vi "Dijkstra.vi"(2 "error in (no error)":errorcluster, 4 "Edges":T1(array[cluster]), 5 "Number of Nodes":i32) -> (0 "error out":errorcluster, 1 "Path":i32[](array[numeric]))   [LabVIEW 2009]
panel:
  out "appended array":dbl[](array[numeric])
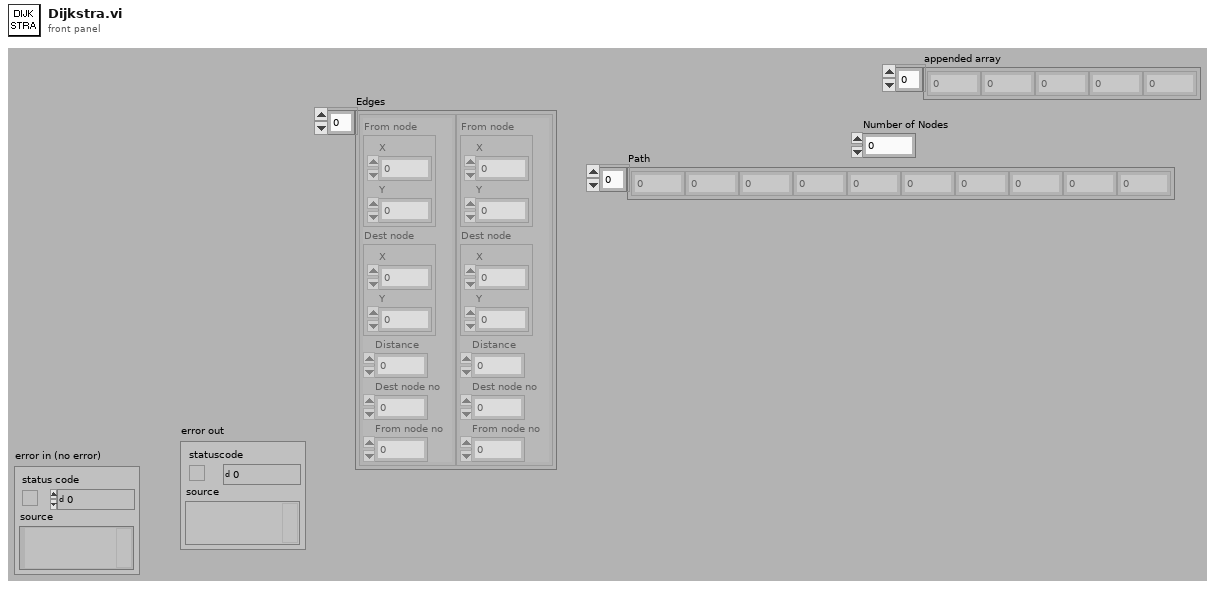
[diagram p1: front panel]
types:
  T1 = cluster{"From node":cluster{"X":dbl, "Y":dbl}, "Dest node":cluster{"X":dbl, "Y":dbl}, "Distance":dbl, "Dest node no":i32, "From node no":i32}[]
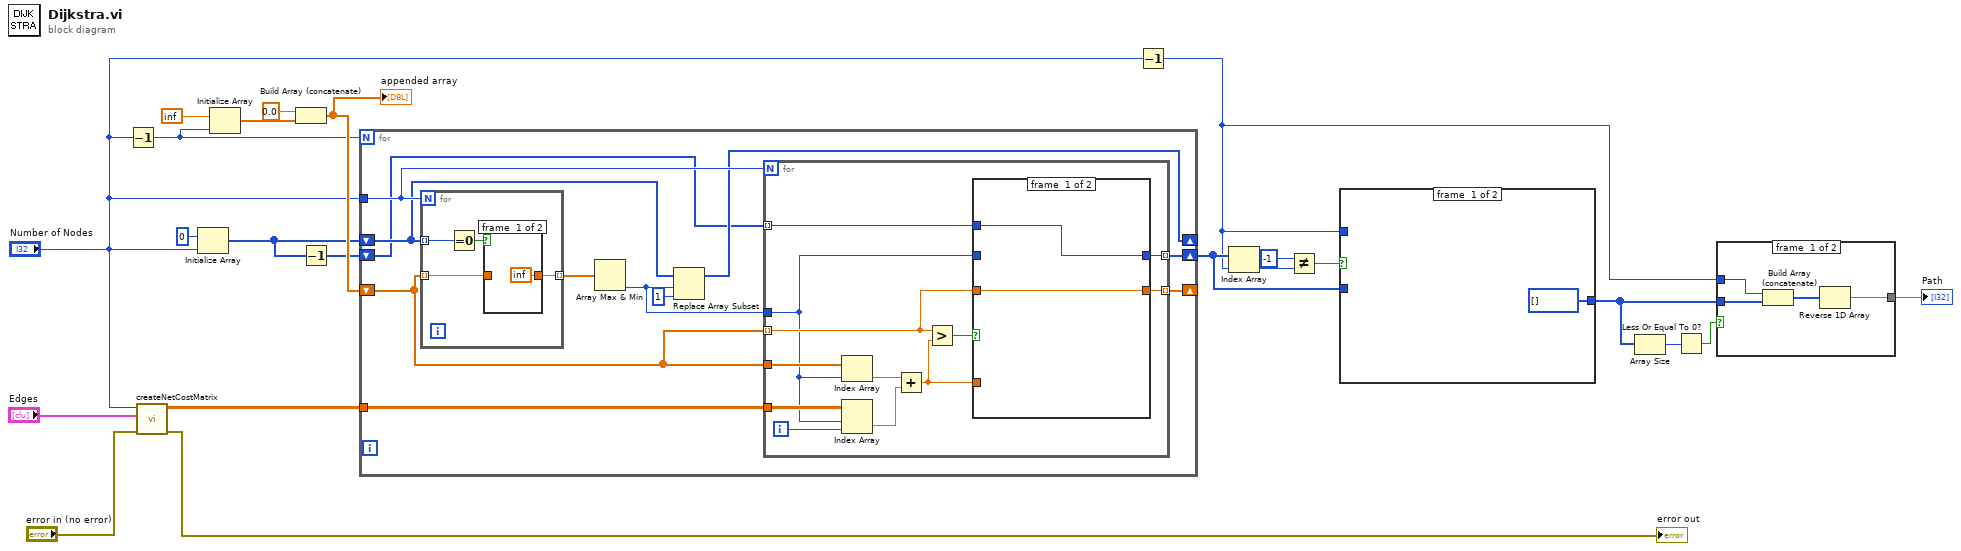
[diagram p0: block diagram]
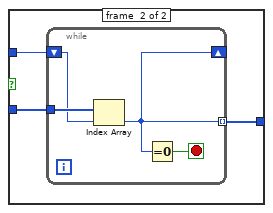
[diagram p3: hidden frame]
diagram:
  n1 = Decrement(x="Number of Nodes") -> (x-1=w10:i32)
  n2 = call "createNetCostMatrix.vi"("error in (no error)"="error in (no error)", "Edges"="Edges", "Number of Nodes"="Number of Nodes") -> ("error out"=→"error out":errorcluster, "netCostMatrix"=w14:dbl[][])  [unwired: 7 in]
  n3 = Initialize Array(0 ("element"), "Number of Nodes") -> (w5:i32[])
  n4 = Initialize Array(inf, w10) -> (w20:dbl[])
  n5 = Build Array (concatenate)(0.0 ("element"), w20) -> (w18:dbl[])
  "appended array" <- w18
  n6 = Decrement(x=w5) -> (x-1=w6:i32[])
  n7 = for {
    N: w10 -> [_]
    tunnel: "Number of Nodes" -> [w32]
    tunnel: w14 -> [w30]
    shift-right: [w25] -> _
    shift-left: w5 -> [w26]
    shift-right: [w27] -> _
    shift-left: w18 -> [w24]
    shift-right: [w28] -> w11
    shift-left: w6 -> [w23]
    n8 = for {
      N: w32 -> [_]
      tunnel: w26 -> [w53] mode=indexing
      tunnel: w24 -> [w51] mode=indexing
      tunnel: [w50] -> w29 mode=indexing
      n9 = Equal To 0?(x=w53) -> (x = 0?=w52:bool)
      n10 = case shown="False" w52 {
        tunnel: w51 -> [_ w55]
        tunnel: [inf w55] -> w50
        frame #0 {
        }
        frame #1 {
        }
      }
    }
    n11 = Array Max & Min(array=w29) -> (min index (indices)=w31:i32)  [unwired: 3 out]
    n12 = Replace Array Subset(array=w26, new element=1 ("new element/subarray"), index=w31) -> (w25:i32[])
    n13 = for {
      N: w32 -> [_]
      tunnel: w31 -> [w36]
      tunnel: w30 -> [w45]
      tunnel: w24 -> [w44]
      tunnel: w24 -> [w39] mode=indexing
      tunnel: w23 -> [w37] mode=indexing
      tunnel: [w35] -> w28 mode=indexing
      tunnel: [w34] -> w27 mode=indexing
      i -> [w42]
      n14 = Index Array(array=w44, index=w36) -> (element=w43:dbl)
      n15 = Index Array(array=w45, index (row)=w36, index (col)=w42) -> (element=w41:dbl)
      n16 = Add(x=w43, y=w41) -> (x+y=w38:dbl)
      n17 = Greater?(x=w39, y=w38) -> (0:w40:bool)
      n18 = case shown="True" w40 {
        tunnel: w39 -> [w47 _]
        tunnel: [w47 w49] -> w34
        tunnel: w38 -> [_ w49]
        tunnel: w37 -> [w46 _]
        tunnel: w36 -> [_ w48]
        tunnel: [w46 w48] -> w35
        frame #0 {
        }
        frame #1 {
        }
      }
    }
  }
  n19 = Decrement(x="Number of Nodes") -> (x-1=w4:i32)
  n20 = Index Array(array=w11, index=w4) -> (element=w13:i32)
  n21 = Not Equal?(x=-1, y=w13) -> (x != y?=w12:bool)
  n22 = case shown="True" w12 {
    tunnel: w4 -> [_ w59]
    tunnel: w11 -> [_ w58]
    tunnel: [i32[] [] w57] -> w3
    frame #0 {
    }
    frame #1 {
      n23 = while {
        shift-right: [w61] -> _
        shift-left: w59 -> [w62]
        tunnel: w58 -> [w63]
        tunnel: [w61] -> w57 mode=indexing
        stop <- w60 stop-if-true
        n24 = Index Array(array=w63, index=w62) -> (element=w61:i32)
        n25 = Equal To 0?(x=w61) -> (x = 0?=w60:bool)
      }
    }
  }
  n26 = Array Size(array=w3) -> (size(s)=w2:i32)
  n27 = Less Or Equal To 0?(x=w2) -> (x <= 0?=w1:bool)
  n28 = case shown="False" w1 {
    tunnel: [w67 w68] -> w8
    tunnel: w4 -> [w65 _]
    tunnel: w3 -> [w64 w68]
    frame #0 {
      n29 = Build Array (concatenate)(w65, w64) -> (w66:i32[])
      n30 = Reverse 1D Array(array=w66) -> (reversed array=w67:i32[])
    }
    frame #1 {
    }
  }
  "Path" <- w8
